vi "test1.vi"() -> ()   [LabVIEW 2019]
panel:
  in  "OK Button":bool
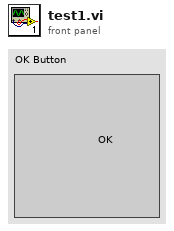
[diagram p1: front panel]
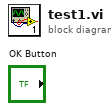
[diagram p0: block diagram]
diagram:
